vi "Run Master.vi"() -> ()   [LabVIEW 2016]
uses:
  <vilib>/NXT/Subs/LVHSConnector.ctl
  <vilib>/NXT/LegoClasses/BrickReference/BrickReference.lvclass
  <vilib>/NXT/Block Support/NXT_ButtonSelector.ctl
  <vilib>/NXT/Dual Mode Library/Waits/Wait_Btn.vi
panel:
  in  "NXT/EV3 in":T1
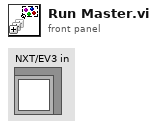
[diagram p1: front panel]
types:
  T1 = typedef "LVHSConnector.ctl" = refnum<class "BrickReference.lvclass">
  T2 = typedef "NXT_ButtonSelector.ctl" = u16
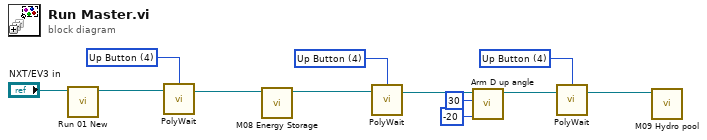
[diagram p0: block diagram]
diagram:
  w1 = T2 4 items=["Enter button"=3, "Left button"=2, "Right button"=1, "Up Button"=4, "Down Button"=5] ("Button (Enter button)")
  w8 = T2 4 items=["Enter button"=3, "Left button"=2, "Right button"=1, "Up Button"=4, "Down Button"=5] ("Button (Enter button)")
  w10 = T2 4 items=["Enter button"=3, "Left button"=2, "Right button"=1, "Up Button"=4, "Down Button"=5] ("Button (Enter button)")
  n1 = call "Run 01 New.vi"("NXT/EV3 in"="NXT/EV3 in") -> ("EV3 out"=w11:T1)  [unwired: 10 in]
  n2 = call-poly <vilib>:"PolyWait.vi"("NXT/EV3"=w11, "Button (Enter button)"=w10) -> ("NXT/EV3"=w9:T1)  [unwired: 2 in]
  n3 = call "M08 Energy Storage.vi"("NXT/EV3"=w9) -> ("EV3 out"=w7:T1)  [unwired: 10 in]
  n4 = call-poly <vilib>:"PolyWait.vi"("NXT/EV3"=w7, "Button (Enter button)"=w8) -> ("NXT/EV3"=w6:T1)  [unwired: 2 in]
  n5 = call "Arm D up angle.vi"("Power"=i8 -20, "Rotation"=30, "EV3 in"=w6) -> ("EV3 out"=w5:T1)  [unwired: 8 in]
  n6 = call-poly <vilib>:"PolyWait.vi"("NXT/EV3"=w5, "Button (Enter button)"=w1) -> ("NXT/EV3"=w2:T1)  [unwired: 2 in]
  n7 = call "M09 Hydro pool.vi"("EV3 in"=w2) -> ()  [unwired: 10 in, 1 out]
